vi "Disconnect Digital Relays.vi"(8 "error in":errorcluster, 11 "TSM context":T1) -> (0 "error out":errorcluster, 3 "TSM context out":T1)   [LabVIEW 2019]
uses:
  <vilib>/NI_TestStand_SemiconductorModule/NI_TestStand_Semiconductor_Module.lvlibp/PinMap/General/SemiconductorModuleContext.ctl
  <instrlib>/niDigital/niDigital.llb/niDigital Selected Function.ctl
  <instrlib>/niDigital/niDigital.llb/niDigital Write Static Pin State.ctl
  Instrument Control/Digital/SSC Digital/Configuration/SSC Digital Select Function.vi
  <vilib>/NI_TestStand_SemiconductorModule/NI_TestStand_Semiconductor_Module.lvlibp
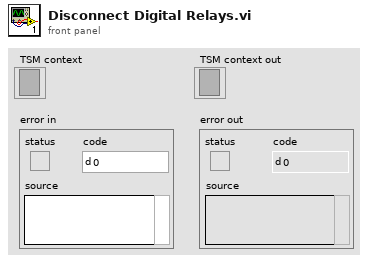
[diagram p1: front panel]
types:
  T1 = typedef "NI_TestStand_Semiconductor_Module.lvlibp/SemiconductorModuleContext.ctl" = refnum<k7>
  T2 = typedef "niDigital Write Static Pin State.ctl" = u8
  T3 = typedef "niDigital Selected Function.ctl" = i32
  T4 = typedef "TSM SSC Digital.ctl" = cluster{"Pin Query Context":refnum<class "DigitalPatternPinQueryContext.lvclass">, "SSC":T5[], "Site Numbers":i32[], "Pins":tag[]}
  T5 = typedef "SSC Digital.ctl" = cluster{"Session":refnum<k15>, "Channel List":string, "Site List":string}
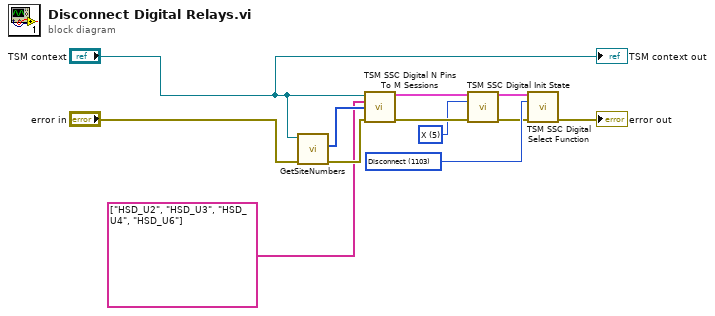
[diagram p0: block diagram]
diagram:
  w8 = T2 5 items=["0"=0, "1"=1, "X"=5] ("state")
  w10 = T3 1103 items=["Digital"=1100, "PPMU"=1101, "Off"=1102, "Disconnect"=1103] ("Select Function")
  n1 = call <vilib>:"GetSiteNumbers.vi"("error in (no error)"="error in", "Semiconductor Module Context"="TSM context") -> ("error out"=w5:errorcluster, "Site Numbers"=w4:i32[])  [unwired: 6 in, 2 out]
  n2 = call "TSM SSC Digital N Pins To M Sessions.vi"("TSM context"="TSM context", "Pins"=tag[] ["HSD_U2", "HSD_U3", "HSD_U4", "HSD_U6"], "Site Numbers"=w4, "error in"=w5) -> ("Digital TSM Out"=w7:T4, "error out"=w12:errorcluster)  [unwired: 10 in]
  n3 = call "TSM SSC Digital Init State.vi"("Digital TSM In"=w7, "state"=w8, "error in"=w12) -> ("Digital TSM Out"=w6:T4, "error out"=w9:errorcluster)  [unwired: 11 in]
  n4 = call "TSM SSC Digital Select Function.vi"("Digital TSM In"=w6, "Function"=w10, "error in"=w9) -> ("error out"=→"error out":errorcluster)  [unwired: 11 in, 1 out]
  "TSM context out" <- "TSM context"
